vi "Calc G,H.vi"(8 "error in (no error)":errorcluster, 10 "End Point":cluster{"X":dbl, "Y":dbl}={"X"=10.0, "Y"=5.0}, 11 "Square In":T1) -> (0 "error out":errorcluster, 2 "Square Out":T1)   [LabVIEW 2009]
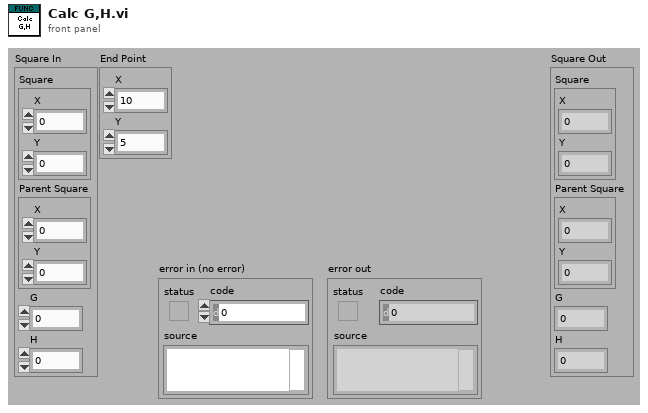
[diagram p1: front panel]
types:
  T1 = cluster{"Square":cluster{"X":dbl, "Y":dbl}, "Parent Square":cluster{"X":dbl, "Y":dbl}, "G":dbl, "H":dbl}
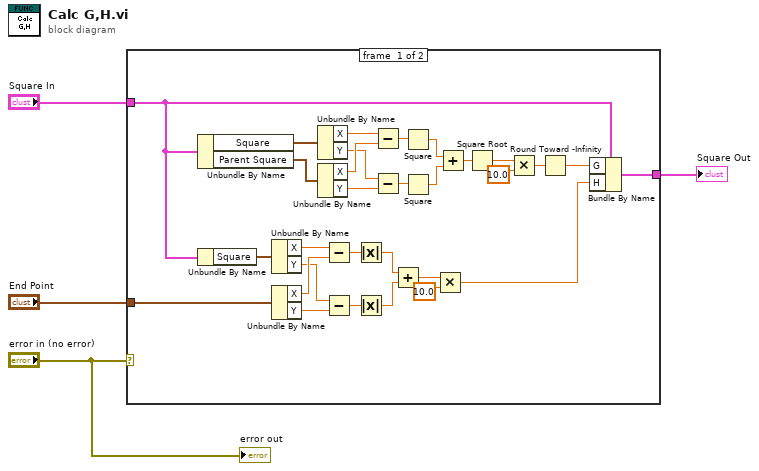
[diagram p0: block diagram]
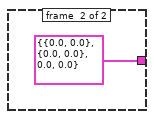
[diagram p2: hidden frame]
diagram:
  n1 = case shown="No Error" "error in (no error)" {
    tunnel: [w22 T1 {"Square"={"X"=0.0, "Y"=0.0}, "Parent Square"={"X"=0.0, "Y"=0.0}, "G"=0.0, "H"=0.0} ("Square In")] -> w4
    tunnel: "End Point" -> [w21 _]
    tunnel: "Square In" -> [w20 _]
    frame #0 {
      n2 = Unbundle By Name(w20) -> ("Square"=w34:cluster{"X":dbl, "Y":dbl}, "Parent Square"=w33:cluster{"X":dbl, "Y":dbl})
      n3 = Unbundle By Name(w20) -> ("Square"=w19:cluster{"X":dbl, "Y":dbl})
      n4 = Unbundle By Name(w19) -> ("X"=w18:dbl, "Y"=w15:dbl)
      n5 = Unbundle By Name(w21) -> ("X"=w16:dbl, "Y"=w17:dbl)
      n6 = Unbundle By Name(w34) -> ("X"=w32:dbl, "Y"=w30:dbl)
      n7 = Unbundle By Name(w33) -> ("X"=w31:dbl, "Y"=w29:dbl)
      n8 = Subtract(x=w18, y=w16) -> (x-y=w14:dbl)
      n9 = Subtract(x=w15, y=w17) -> (x-y=w13:dbl)
      n10 = Absolute Value(x=w14) -> (abs(x)=w9:dbl)
      n11 = Absolute Value(x=w13) -> (abs(x)=w8:dbl)
      n12 = Subtract(x=w32, y=w31) -> (x-y=w28:dbl)
      n13 = Subtract(x=w30, y=w29) -> (x-y=w27:dbl)
      n14 = Add(x=w9, y=w8) -> (x+y=w6:dbl)
      n15 = Square(x=w28) -> (x^2=w26:dbl)
      n16 = Square(x=w27) -> (x^2=w25:dbl)
      n17 = Multiply(x=w6, y=10.0) -> (x*y=w5:dbl)
      n18 = Add(x=w26, y=w25) -> (x+y=w24:dbl)
      n19 = Square Root(x=w24) -> (sqrt(x)=w12:dbl)
      n20 = Multiply(x=w12, y=10.0) -> (x*y=w10:dbl)
      n21 = Round Toward -Infinity(1:w10) -> (0:w23:dbl)
      n22 = Bundle By Name(cluster=w20, "G"=w23, "H"=w5) -> (w22:T1)
    }
    frame #1 {
    }
  }
  "Square Out" <- w4
  "error out" <- "error in (no error)"
